vi "SeparaMemoriaPlayRotacao.vi"(8 "error in":errorcluster, 11 "Acionamento":enum16{"Play", "Stop"}(ring)) -> (0 "error out":errorcluster, 2 "InfoStatus":string, 3 "Memorias":T1(array[cluster]))   [LabVIEW 2019]
uses:
  TelaConfig/Configuracao.Variaveis.vi
  VariaveisMedicao.vi
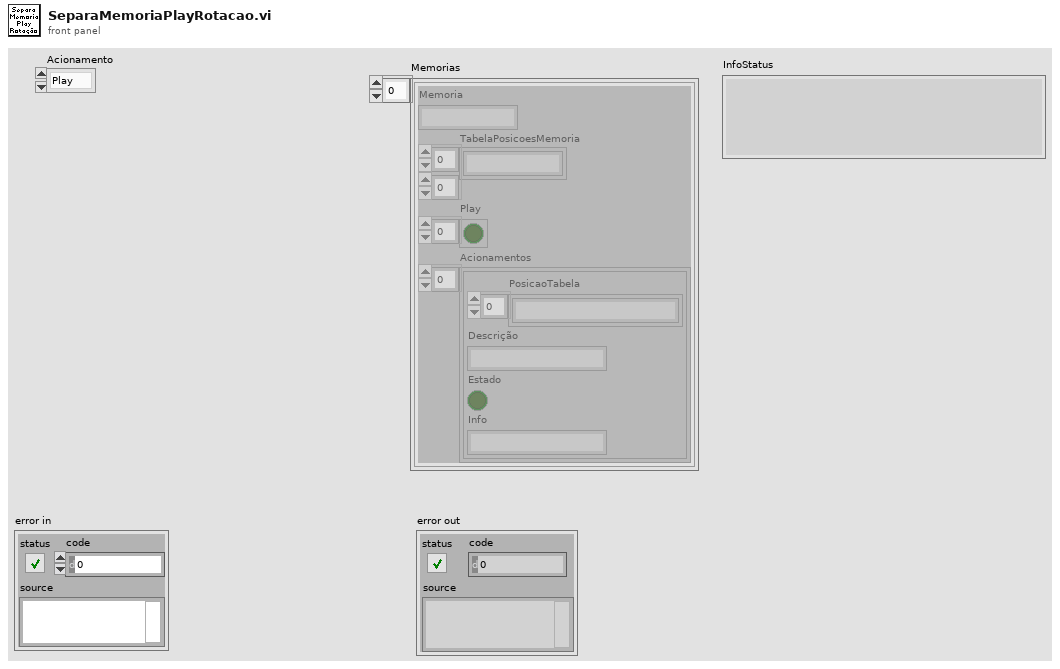
[diagram p1: front panel]
types:
  T1 = cluster{"Memoria":string, "TabelaPosicoesMemoria":string[][], "Play":bool[], "Acionamentos":cluster{"PosicaoTabela":string[], "Descrição":string, "Estado":bool, "Info":string}[]}[]
  T2 = cluster{"Memoria":string, "TabelaPosicoesMemoria":string[][]}[]
  T3 = cluster{"Acionamento":string, "Descrição":string, "Info True":string, "Info False":string, "Play":bool}[]
  T4 = cluster{"Memoria":string, "TabelaPosicoesMemoria":string[][]}
  T5 = cluster{"Memoria":string, "TabelaPosicoesMemoria":string[][], "Play":bool[], "Acionamentos":cluster{"PosicaoTabela":string[], "Descrição":string, "Estado":bool, "Info":string}[]}
  T6 = cluster{"PosicaoTabela":string[], "Descrição":string, "Estado":bool, "Info":string}
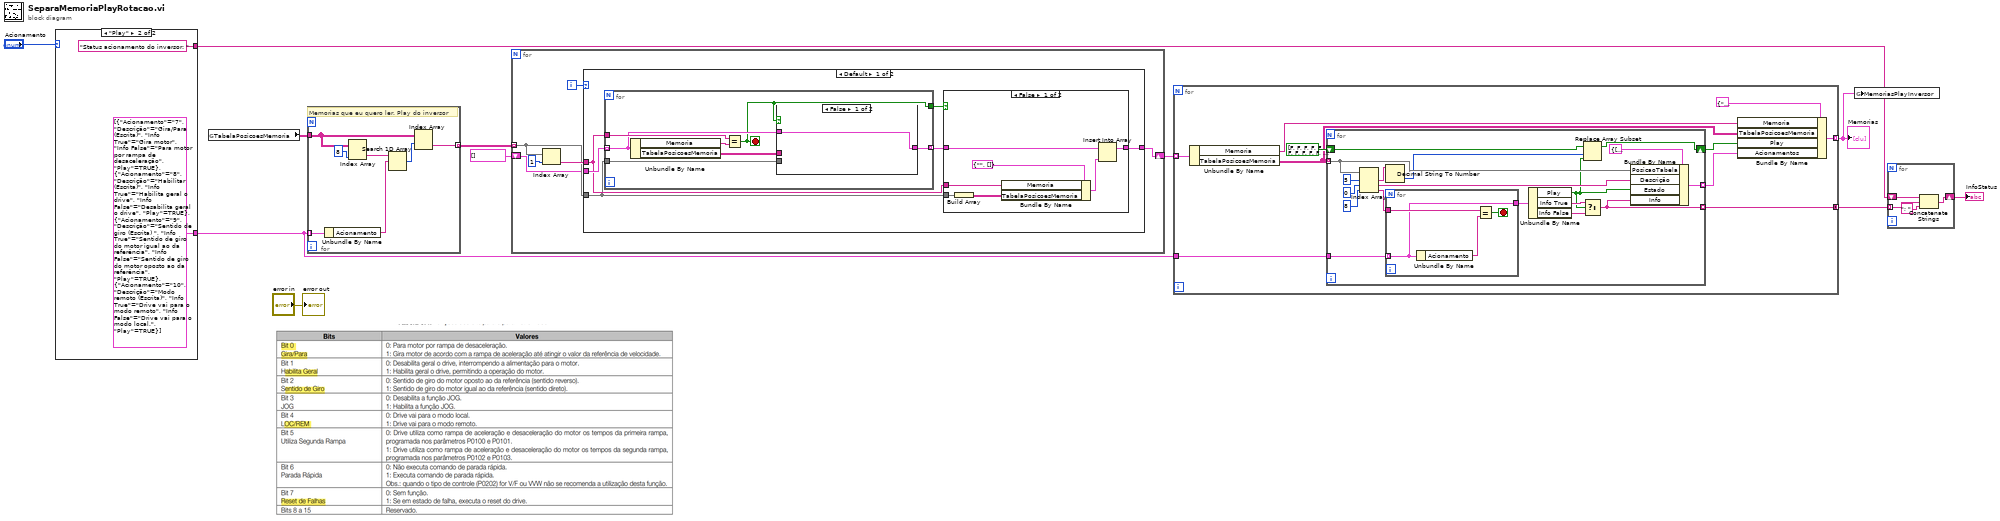
[diagram p0: block diagram]
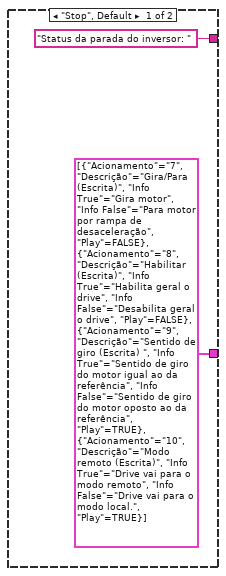
[diagram p2: hidden frame]
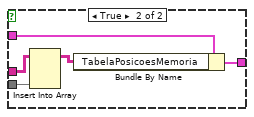
[diagram p4: hidden frame]
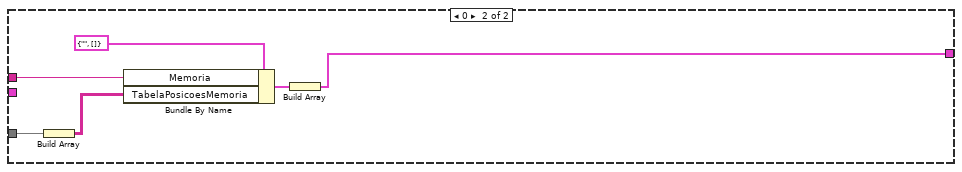
[diagram p5: hidden frame]
diagram:
  n1 = case shown="\"Play\"" "Acionamento" {
    tunnel: [T3 [{"Acionamento"="7", "Descrição"="Gira/Para (Escrita)", "Info True"="Gira motor", "Info False"="Para motor por rampa de desaceleração", "Play"=FALSE}, {"Acionamento"="8", "Descrição"="Habilitar (Escrita)", "Info True"="Habilita geral o drive", "Info False"="Desabilita geral o drive", "Play"=FALSE}, {"Acionamento"="9", "Descrição"="Sentido de giro (Escrita) ", "Info True"="Sentido de giro do motor igual ao da referência", "Info False"="Sentido de giro do motor oposto ao da referência", "Play"=TRUE}, {"Acionamento"="10", "Descrição"="Modo remoto (Escrita)", "Info True"="Drive vai para o modo remoto", "Info False"="Drive vai para o modo local.", "Play"=TRUE}] ("Array") T3 [{"Acionamento"="7", "Descrição"="Gira/Para (Escrita)", "Info True"="Gira motor", "Info False"="Para motor por rampa de desaceleração", "Play"=TRUE}, {"Acionamento"="8", "Descrição"="Habilitar (Escrita)", "Info True"="Habilita geral o drive", "Info False"="Desabilita geral o drive", "Play"=TRUE}, {"Acionamento"="9", "Descrição"="Sentido de giro (Escrita) ", "Info True"="Sentido de giro do motor igual ao da referência", "Info False"="Sentido de giro do motor oposto ao da referência", "Play"=TRUE}, {"Acionamento"="10", "Descrição"="Modo remoto (Escrita)", "Info True"="Drive vai para o modo remoto", "Info False"="Drive vai para o modo local.", "Play"=TRUE}] ("Array")] -> w2
    tunnel: ["Status da parada do inversor: " "Status acionamento do inversor: "] -> w5
    frame "Stop", Default {
    }
    frame "Play" {
    }
  }
  n2 = global read "Configuracao.Variaveis.vi" "TabelaPosicoesMemoria"() -> (w10:string[][])
  n3 = for {
    tunnel: w10 -> [w19]
    tunnel: [w18] -> w11 mode=indexing
    tunnel: w2 -> [w17] mode=indexing
    # "Memorias que eu quero ler. Play do inversor"
    n4 = Unbundle By Name(w17) -> ("Acionamento"=w16:string)
    n5 = Index Array(array=w19, index (col)=8 ("disabled index (col)")) -> (element=w20:string[])  [unwired: 1 in]
    n6 = Search 1D Array(1D array=w20, element=w16) -> (index of element=w22:i32)  [unwired: 1 in]
    n7 = Index Array(array=w19, index (row)=w22) -> (element=w18:string[])  [unwired: 1 in]
  }
  n8 = for {
    tunnel: w11 -> [w25] mode=indexing
    shift-right: [w24] -> w7
    shift-left: T2 [] ("Memorias") -> [w23]
    i -> [w27]
    n9 = Index Array(array=w25, index=1) -> (element=w26:string)
    n10 = case shown="Default" w27 {
      tunnel: w26 -> [w30 w61]
      tunnel: w25 -> [w29 w60]
      tunnel: [w32 w57] -> w24
      tunnel: w23 -> [w34 _]
      frame Default {
        n11 = for {
          tunnel: w34 -> [w47] mode=indexing
          tunnel: w30 -> [w48]
          tunnel: w29 -> [w45]
          tunnel: [w44] -> w31 mode=indexing
          tunnel: [w43] -> w33
          stop <- w43 stop-if-true
          n12 = Unbundle By Name(w47) -> ("Memoria"=w49:string, "TabelaPosicoesMemoria"=w46:string[][])
          n13 = Equal?(x=w48, y=w49) -> (x = y?=w43:bool)
          n14 = case shown="False" w43 {
            tunnel: w47 -> [w50 w55]
            tunnel: w46 -> [_ w54]
            tunnel: w45 -> [_ w53]
            tunnel: [w50 w51] -> w44
            frame False {
            }
            frame True {
              n15 = Insert Into Array(array=w54, new element=w53) -> (w52:string[][])  [unwired: 2 in]
              n16 = Bundle By Name(cluster=w55, "TabelaPosicoesMemoria"=w52) -> (w51:T4)
            }
          }
        }
        n17 = case shown="False" w33 {
          tunnel: [w36 w42] -> w32
          tunnel: w31 -> [w38 w42]
          tunnel: w30 -> [w41 _]
          tunnel: w29 -> [w40 _]
          frame False {
            n18 = Build Array(w40) -> (w39:string[][])
            n19 = Bundle By Name(cluster=T4 {"Memoria"="", "TabelaPosicoesMemoria"=[]} ("Cluster"), "Memoria"=w41, "TabelaPosicoesMemoria"=w39) -> (w37:T4)
            n20 = Insert Into Array(array=w38, new element=w37) -> (w36:T2)  [unwired: 1 in]
          }
          frame True {
          }
        }
      }
      frame 0 {
        n21 = Build Array(w60) -> (w59:string[][])
        n22 = Bundle By Name(cluster=T4 {"Memoria"="", "TabelaPosicoesMemoria"=[]} ("Cluster"), "Memoria"=w61, "TabelaPosicoesMemoria"=w59) -> (w58:T4)
        n23 = Build Array(w58) -> (w57:T2)
      }
    }
  }
  n24 = for {
    tunnel: w7 -> [w71] mode=indexing
    tunnel: w2 -> [w68]
    tunnel: [w63] -> w1 mode=indexing
    tunnel: [w62] -> w4 mode=concatenating
    n25 = Unbundle By Name(w71) -> ("Memoria"=w69:string, "TabelaPosicoesMemoria"=w66:string[][])
    n26 = for {
      tunnel: [w86] -> w64 mode=indexing
      tunnel: w66 -> [w84] mode=indexing
      tunnel: w68 -> [w82]
      shift-right: [w77] -> w65
      shift-left: bool[] [FALSE, FALSE, FALSE, FALSE, FALSE, FALSE, FALSE, FALSE, FALSE, FALSE, FALSE, FALSE, FALSE, FALSE, FALSE] ("Array 2") -> [w80]
      tunnel: [w72] -> w62 mode=indexing
      n27 = Index Array(array=w84, index #1=5 ("index"), index #2=0 ("index"), index #3=8 ("index")) -> (element #1=w88:string, element #2=w74:string, element #3=w83:string)
      n28 = Decimal String To Number(string=w88) -> (number=w78:i32)  [unwired: 2 in, 1 out]
      n29 = for {
        tunnel: w83 -> [w92]
        tunnel: w82 -> [w90] mode=indexing
        tunnel: [w90] -> w79
        stop <- w91 stop-if-true
        n30 = Unbundle By Name(w90) -> ("Acionamento"=w93:string)
        n31 = Equal?(x=w92, y=w93) -> (x = y?=w91:bool)
      }
      n32 = Unbundle By Name(w79) -> ("Play"=w73:bool, "Info True"=w76:string, "Info False"=w75:string)
      n33 = Replace Array Subset(array=w80, new element=w73, index=w78) -> (w77:bool[])
      n34 = Select(t=w76, s=w73, f=w75) -> (s? t:f=w72:string)
      n35 = Bundle By Name(cluster=T6 {"PosicaoTabela"=[], "Descrição"="", "Estado"=FALSE, "Info"=""} ("Cluster"), "PosicaoTabela"=w84, "Descrição"=w74, "Estado"=w73, "Info"=w72) -> (w86:T6)
    }
    n36 = Bundle By Name(cluster=T5 {"Memoria"="", "TabelaPosicoesMemoria"=[], "Play"=[], "Acionamentos"=[]} ("Cluster"), "Memoria"=w69, "TabelaPosicoesMemoria"=w66, "Play"=w65, "Acionamentos"=w64) -> (w63:T5)
  }
  "Memorias" <- w1
  n37 = global write "VariaveisMedicao.vi" "MemoriasPlayInversor"(w1) -> ()
  n38 = for {
    shift-right: [w95] -> w3
    shift-left: w5 -> [w97]
    tunnel: w4 -> [w96] mode=indexing
    n39 = Concatenate Strings(w97, w96, "; " ("string")) -> (w95:string)
  }
  "InfoStatus" <- w3
  "error out" <- "error in"
